vi "265_data.vi"() -> ()   [LabVIEW 2020]
panel:
  out "x/y":dbl
  out "x+y 2":timestamp format="%<%.8X\n%x>T"
  out "x+y":timestamp format="%<%.8X\n%x>T"
  out "x-y 6":u64
  out "x-y 5":u64
  out "x-y 4":u64
  out "x-y 3":u64
  out "x-y 2":u64
  out "x-y":u64
  out "TDMS LLP 2K Frist Frame":u64
  out "TDMS LLP 4K First Frame":u64
  out "TDMS CANLOG Time Stamp (ns)":u64
  in  "TDMS CANLOG Time Stamp":timestamp=timestamp(3761638239.819426 s since 1904-01-01) format="%<%.6X\n%x>T"
  out "2k First Frame":timestamp format="%<%.8X\n%x>T"
  out "2k First Frame (ns)":u64=1676028445810222898
  out "4k First Frame (ns)":u64=1676028445810222898
  out "CAN First Frame (ns)":u64
  out "4k First Frame":timestamp format="%<%.9X\n%x>T"
  out "CAN First Frame":timestamp format="%<%.8X\n%x>T"
  in  "Time Stamp":timestamp=timestamp(3758873160.511 s since 1904-01-01)
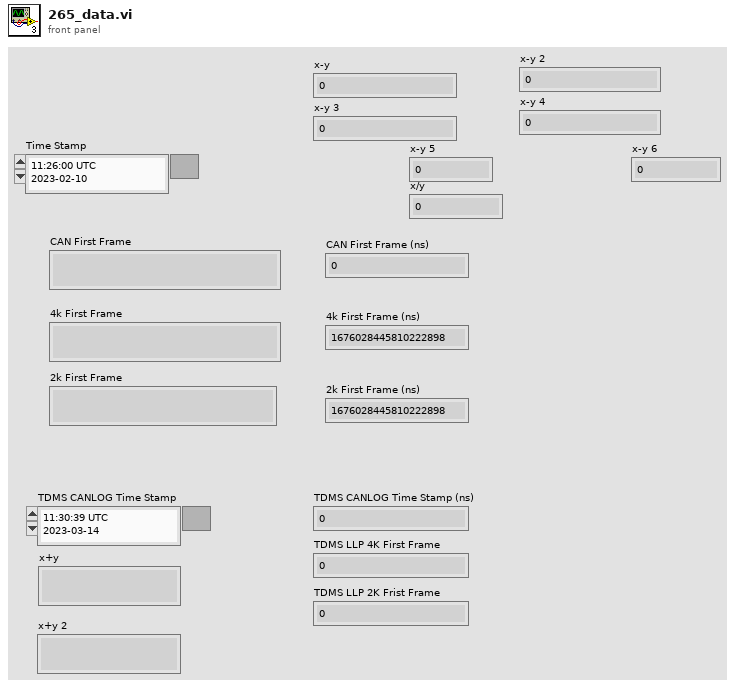
[diagram p1: front panel]
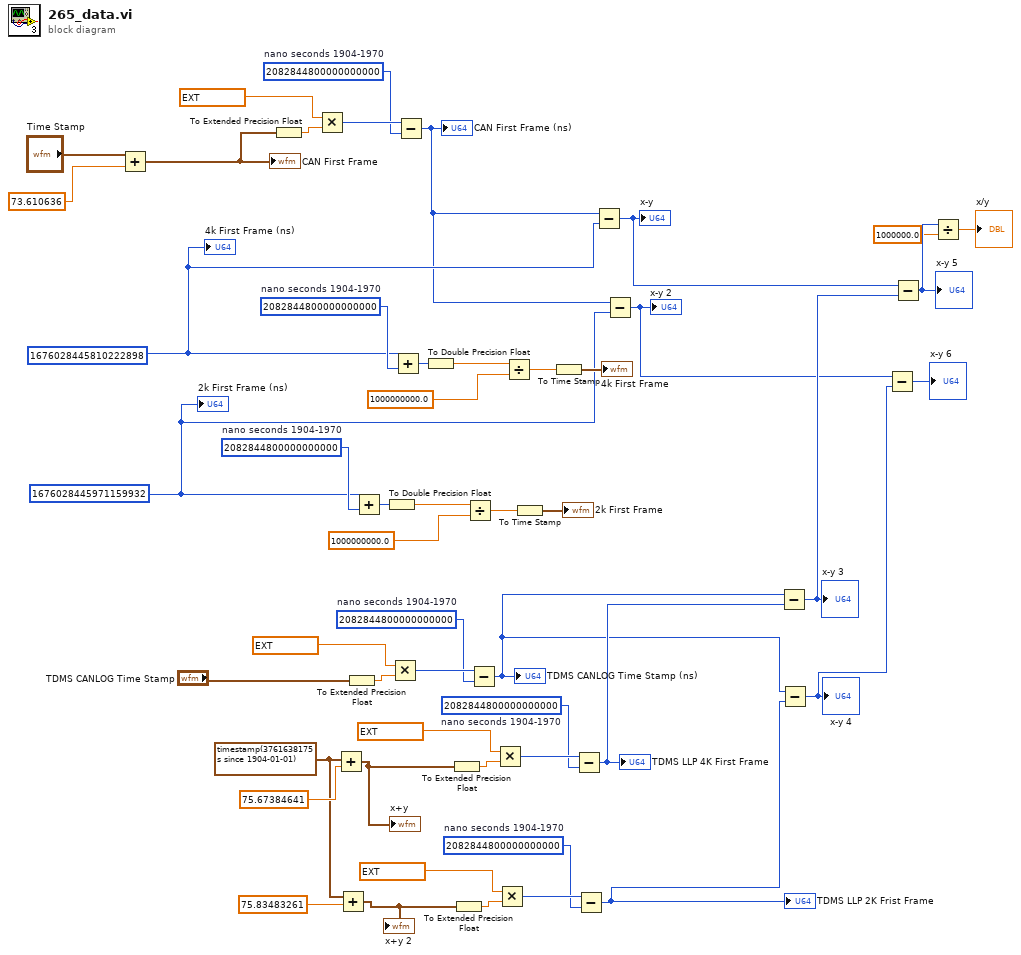
[diagram p0: block diagram]
diagram:
  w19 = u64 2082844800000000000  # nano seconds 1904-1970
  w24 = u64 2082844800000000000  # nano seconds 1904-1970
  w15 = timestamp(3761638175.834725 s since 1904-01-01) ("TDMS CANLOG Time Stamp")
  w30 = u64 2082844800000000000  # nano seconds 1904-1970
  w38 = u64 2082844800000000000  # nano seconds 1904-1970
  w12 = u64 1676028445971159932
  w41 = u64 2082844800000000000  # nano seconds 1904-1970
  w49 = u64 2082844800000000000  # nano seconds 1904-1970
  w14 = u64 1676028445810222898
  n1 = Add(x="Time Stamp", y=73.610636) -> (x+y=w40:timestamp)
  "CAN First Frame" <- w40
  n2 = To Extended Precision Float(1:w40) -> (0:w43:ext)
  n3 = Multiply(x=ext 1000000000.0, y=w43) -> (x*y=w42:u64)
  n4 = Add(x=w15, y=75.67384641) -> (x+y=w22:timestamp)
  "x+y" <- w22
  n5 = Add(x=w15, y=75.83483261) -> (x+y=w17:timestamp)
  "x+y 2" <- w17
  n6 = To Extended Precision Float(1:"TDMS CANLOG Time Stamp") -> (0:w32:ext)
  n7 = Add(x=w12, y=w38) -> (x+y=w37:u64)
  n8 = To Double Precision Float(number=w37) -> (double precision float=w36:dbl)
  n9 = Multiply(x=ext 1000000000.0, y=w32) -> (x*y=w31:u64)
  n10 = Add(x=w14, y=w49) -> (x+y=w48:u64)
  n11 = Subtract(x=w42, y=w41) -> (x-y=w13:u64)
  "CAN First Frame (ns)" <- w13
  n12 = To Double Precision Float(number=w48) -> (double precision float=w47:dbl)
  n13 = To Extended Precision Float(1:w22) -> (0:w26:ext)
  n14 = To Extended Precision Float(1:w17) -> (0:w21:ext)
  n15 = Divide(x=w36, y=1000000000.0) -> (x/y=w34:dbl)
  n16 = Subtract(x=w31, y=w30) -> (x-y=w10:u64)
  "TDMS CANLOG Time Stamp (ns)" <- w10
  n17 = Multiply(x=ext 1000000000.0, y=w26) -> (x*y=w25:u64)
  n18 = Multiply(x=ext 1000000000.0, y=w21) -> (x*y=w20:u64)
  n19 = Divide(x=w47, y=1000000000.0) -> (x/y=w45:dbl)
  n20 = To Time Stamp(1:w34) -> (0:→"2k First Frame":timestamp)
  n21 = To Time Stamp(1:w45) -> (0:→"4k First Frame":timestamp)
  n22 = Subtract(x=w25, y=w24) -> (x-y=w11:u64)
  "TDMS LLP 4K First Frame" <- w11
  n23 = Subtract(x=w20, y=w19) -> (x-y=w9:u64)
  "TDMS LLP 2K Frist Frame" <- w9
  n24 = Subtract(x=w13, y=w14) -> (x-y=w8:u64)
  "x-y" <- w8
  n25 = Subtract(x=w13, y=w12) -> (x-y=w6:u64)
  "x-y 2" <- w6
  n26 = Subtract(x=w10, y=w11) -> (x-y=w7:u64)
  "x-y 3" <- w7
  n27 = Subtract(x=w10, y=w9) -> (x-y=w5:u64)
  "x-y 4" <- w5
  n28 = Subtract(x=w6, y=w5) -> (x-y=→"x-y 6":u64)
  n29 = Subtract(x=w8, y=w7) -> (x-y=w3:u64)
  "x-y 5" <- w3
  n30 = Divide(x=w3, y=1000000.0) -> (x/y=→"x/y":dbl)
  "4k First Frame (ns)" <- w14
  "2k First Frame (ns)" <- w12
